vi "Get Board Info From Installed.vi"() -> (1 "Sorted ID":u32[](array[numeric]), 2 "Sorted Fam":u32[](array[numeric]), 3 "Sorted name":string[](array[string]))   [LabVIEW 2019, in "LINXx.lvlib"]
doc: "Get family/IDs from installed LINX library"
uses:
  LINXx.lvlib
  <vilib>/regexp/Match Regular Expression.xnode
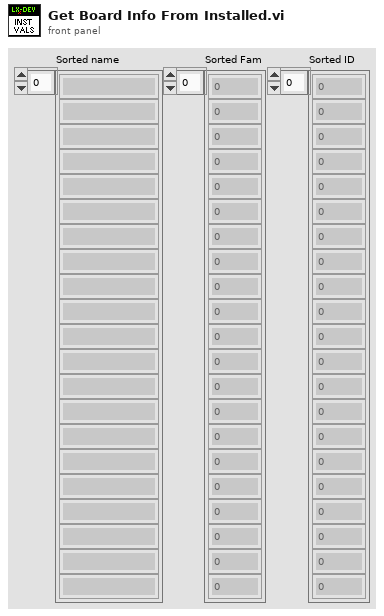
[diagram p1: front panel]
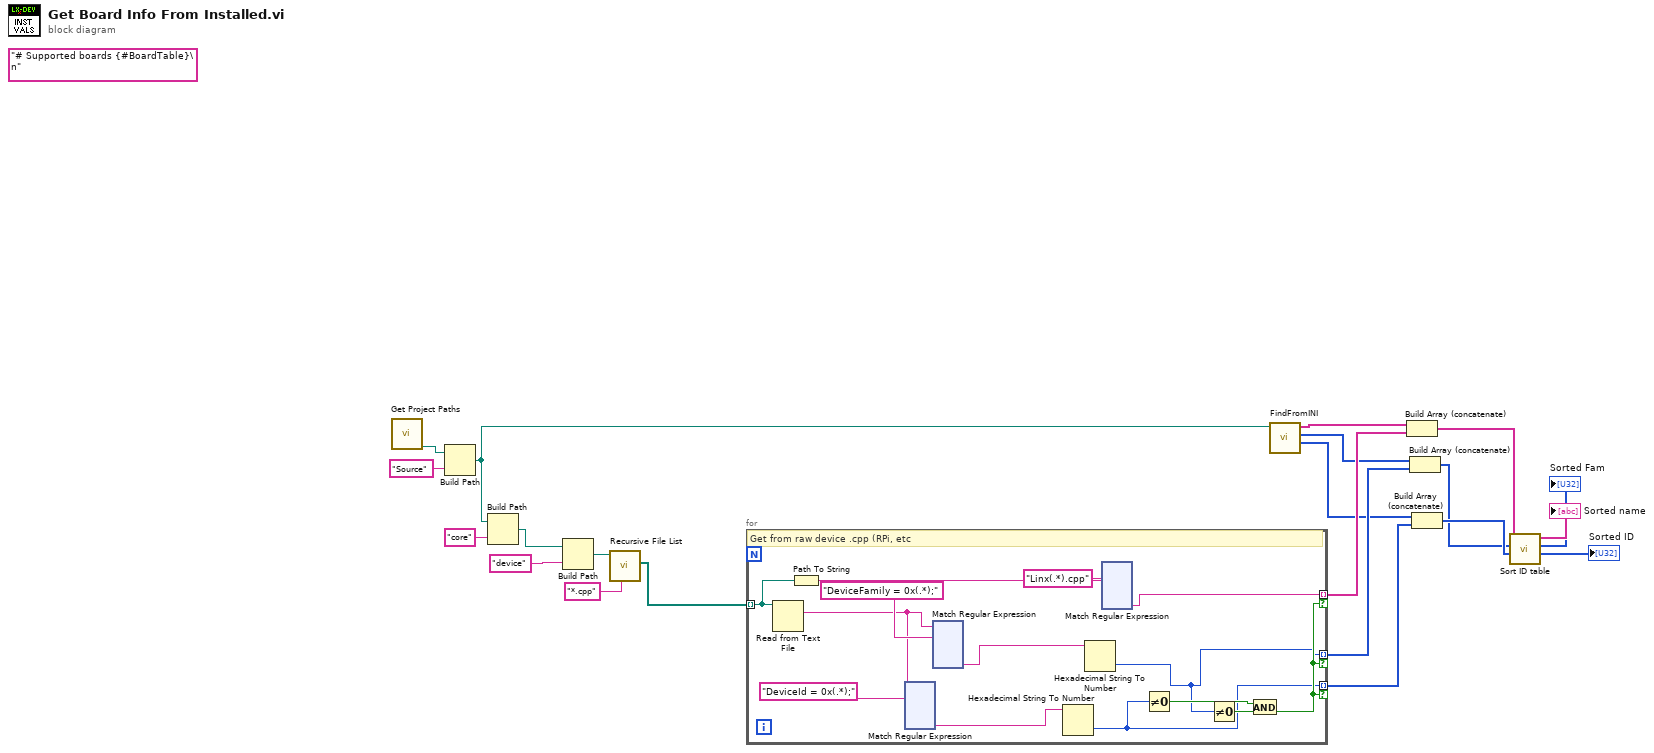
[diagram p0: block diagram]
diagram:
  (unwired) "# Supported boards {#BoardTable}\n"
  n1 = call "Get Project Paths.vi"() -> ("Installed FW path"=w20:path)  [unwired: 8 in, 3 out]
  n2 = Build Path(base path=w20, name or relative path="Source") -> (appended path=w18:path)
  n3 = Build Path(base path=w18, name or relative path="core") -> (appended path=w15:path)
  n4 = Build Path(base path=w15, name or relative path="device") -> (appended path=w14:path)
  n5 = call <vilib>:"Recursive File List.vi"("pattern"="*.cpp", "Folder Path"=w14) -> ("All Files in Dir"=w13:path[])  [unwired: 5 in, 4 out]
  n6 = for {
    tunnel: [w22] -> w7 mode=indexing if=w25
    tunnel: [w23] -> w8 mode=indexing if=w25
    tunnel: w13 -> [w28] mode=indexing
    tunnel: [w29] -> w6 mode=indexing if=w25
    # "Get from raw device .cpp (RPi, etc"
    n7 = Read from Text File(file (use dialog)=w28) -> (text=w31:string)  [unwired: 3 in, 3 out]
    n8 = Path To String(path=w28) -> (string=w27:string)
    n9 = xnode "Match Regular Expression"("input string"=w31, "regular expression"="DeviceId = 0x(.*);") -> ("submatch 1"=w33:string)  [unwired: 4 in, 5 out]
    n10 = xnode "Match Regular Expression"("input string"=w31, "regular expression"="DeviceFamily = 0x(.*);") -> ("submatch 1"=w32:string)  [unwired: 4 in, 5 out]
    n11 = Hexadecimal String To Number(string=w33) -> (number=w23:u32)  [unwired: 2 in, 1 out]
    n12 = Hexadecimal String To Number(string=w32) -> (number=w22:u32)  [unwired: 2 in, 1 out]
    n13 = xnode "Match Regular Expression"("input string"=w27, "regular expression"="Linx(.*).cpp") -> ("submatch 1"=w29:string)  [unwired: 4 in, 5 out]
    n14 = Not Equal To 0?(x=w23) -> (x != 0?=w24:bool)
    n15 = Not Equal To 0?(x=w22) -> (x != 0?=w26:bool)
    n16 = And(x=w24, y=w26) -> (x .and. y?=w25:bool)
  }
  n17 = call "FindFromINI.vi"("INI folder"=w18) -> ("IDs"=w4:u32[], "Families"=w5:u32[], "Names"=w9:string[])  [unwired: 7 in, 1 out]
  n18 = Build Array (concatenate)(w9, w6) -> (w1:string[])
  n19 = Build Array (concatenate)(w5, w7) -> (w2:u32[])
  n20 = Build Array (concatenate)(w4, w8) -> (w3:u32[])
  n21 = call "Sort ID table.vi"("ID"=w3, "Family"=w2, "Name"=w1) -> ("Sorted ID"=→"Sorted ID":u32[], "Sorted Fam"=→"Sorted Fam":u32[], "Sorted name"=→"Sorted name":string[])  [unwired: 6 in]
